vi "Rabi Pulse.vi"() -> ()   [LabVIEW 2012]
uses:
  <vilib>/DAQmx/read.llb/DAQmx Read (Digital Bool 1Line 1Point).vi
  <vilib>/Utility/file.llb/Write To Spreadsheet File (DBL).vi
  <vilib>/DAQmx/create/channels.llb/DAQmx Create Channel (DI-Digital Input).vi
  <vilib>/DAQmx/miscellaneous.llb/DAQmx Fill In Error Info.vi
panel:
  out "Run":bool
  out "size(s)":i32=225
  in  "file path (dialog if empty)":path=path "C:/Users/Ouyang Group/Documents/Data/12-5-13/Rabi pulse sequence 7"
  in  "AOM Pulse length":dbl=3e-07
  in  "N Loop":i32=25000
  in  "Path to spinapi.dll":path=path "C:/SpinCore/SpinAPI/dll/spinapi64.dll"
  in  "stop":bool
  in  "start/restart":bool
  in  "MW width Max":dbl=5e-07
  in  "MW width step size":dbl=2e-09
  in  "MW width Min":dbl=5e-08
  in  "clock_freq (MHz)":dbl=300.0
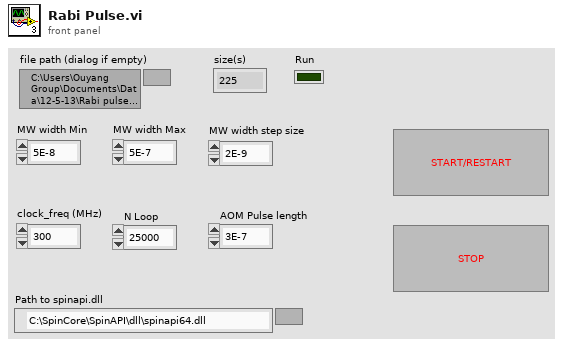
[diagram p1: front panel]
types:
  T1 = cluster{"Instruct Data":i32, "Op Code":i32, "Flags":bool[], "Comments":string, "Time (s)":dbl}
  T2 = enum16{"Pulse Program", "Frequency Registers", "TX Phase Registers", "RX Phase Registers"}
  T3 = cluster{"Instruct Data":i32, "Op Code":i32, "Flags":bool[], "Comments":string, "Time (s)":dbl}[]
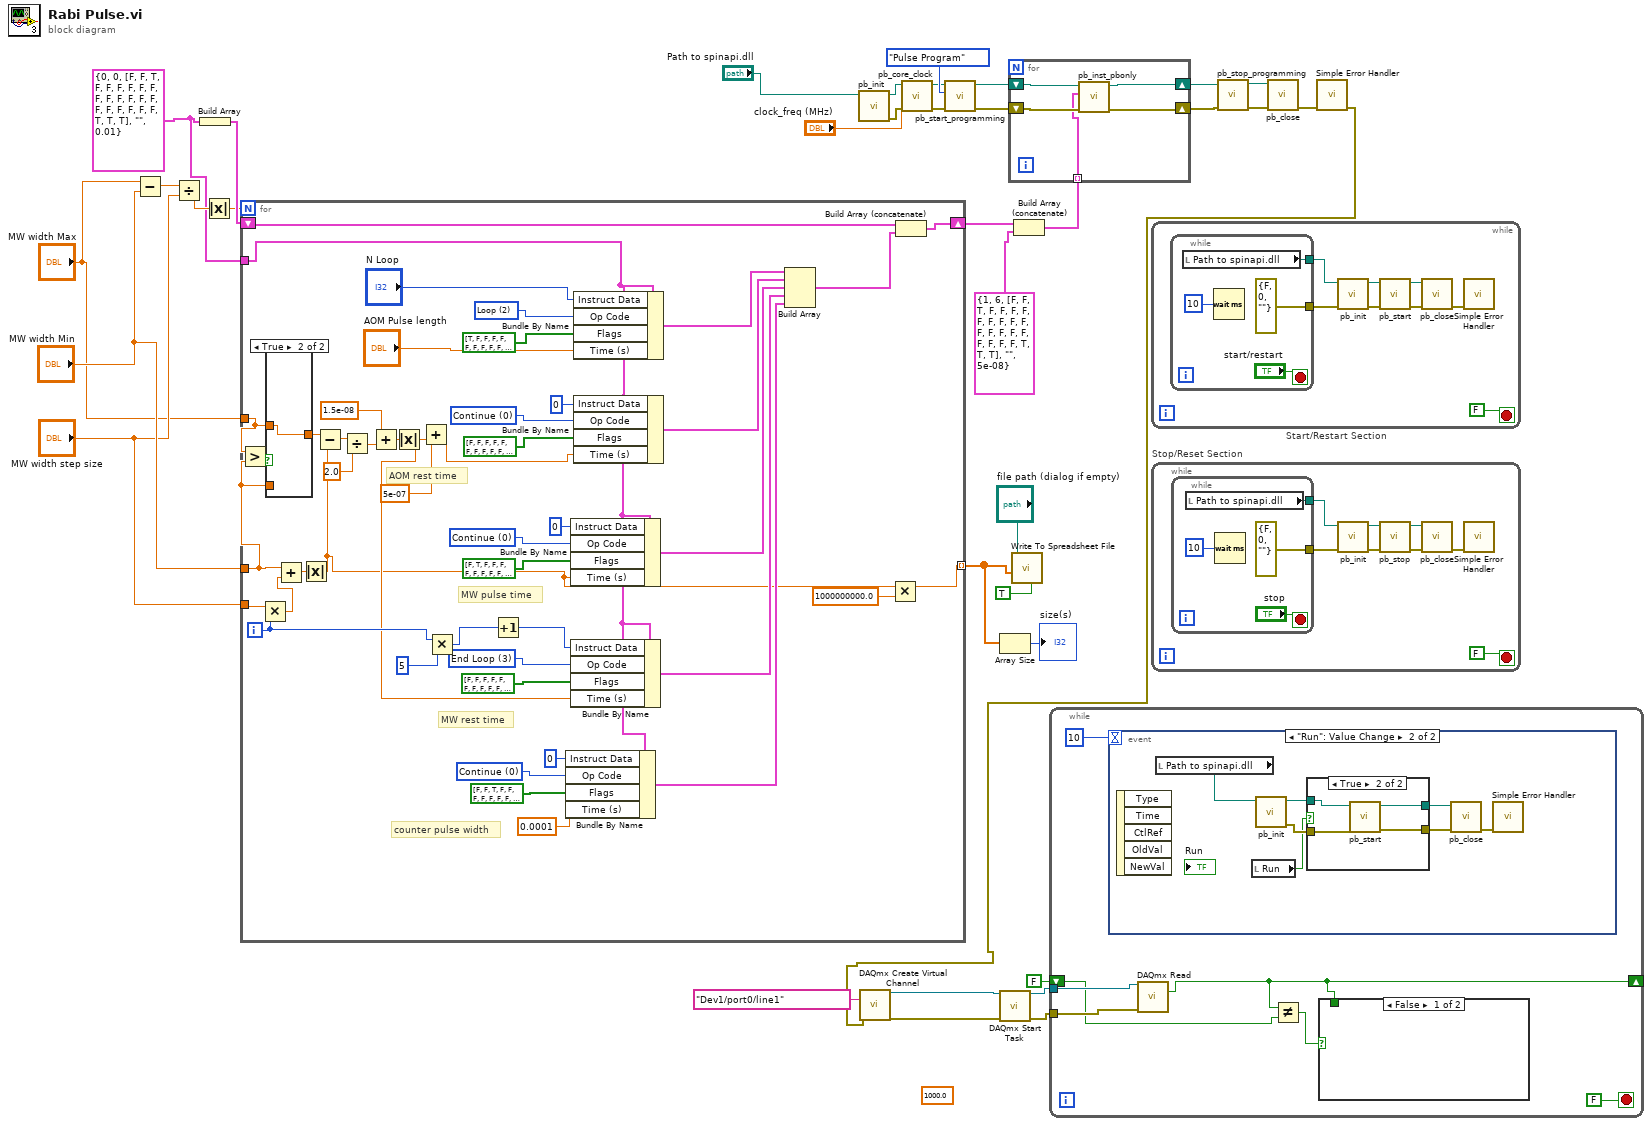
[diagram p0: block diagram]
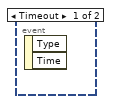
[diagram p2: hidden frame]
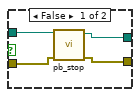
[diagram p3: hidden frame]
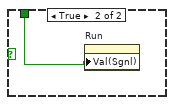
[diagram p4: hidden frame]
diagram:
  (unwired) 1000.0 ("rate")
  w20 = T1 {"Instruct Data"=0, "Op Code"=0, "Flags"=[FALSE, FALSE, TRUE, FALSE, FALSE, FALSE, FALSE, FALSE, FALSE, FALSE, FALSE, FALSE, FALSE, FALSE, FALSE, FALSE, FALSE, FALSE, FALSE, FALSE, FALSE, TRUE, TRUE, TRUE], "Comments"="", "Time (s)"=0.01} ("PB Inst 2")
  n1 = Subtract(x="MW width Max", y="MW width Min") -> (x-y=w24:dbl)
  n2 = Divide(x=w24, y="MW width step size") -> (x/y=w23:dbl)
  n3 = Build Array(w20) -> (w19:T3)
  n4 = Absolute Value(x=w23) -> (abs(x)=w1:dbl)
  n5 = for {
    N: w1 -> [_]
    tunnel: "MW width Min" -> [w39]
    tunnel: "MW width step size" -> [w83]
    tunnel: [w52] -> w11 mode=indexing
    tunnel: w20 -> [w56]
    shift-right: [w80] -> w18
    shift-left: w19 -> [w81]
    tunnel: "MW width Max" -> [w40]
    i -> [w53]
    w67 = 0 items=["Continue", "Stop", "Loop", "End Loop", "JSR", "RTS", "Branch", "Long Delay", "Wait"] ("Op Code")
    w69 = 3 items=["Continue", "Stop", "Loop", "End Loop", "JSR", "RTS", "Branch", "Long Delay", "Wait"] ("Op Code")
    w72 = 0 items=["Continue", "Stop", "Loop", "End Loop", "JSR", "RTS", "Branch", "Long Delay", "Wait"] ("Op Code")
    w75 = 0 items=["Continue", "Stop", "Loop", "End Loop", "JSR", "RTS", "Branch", "Long Delay", "Wait"] ("Op Code")
    w78 = 2 items=["Continue", "Stop", "Loop", "End Loop", "JSR", "RTS", "Branch", "Long Delay", "Wait"] ("Op Code")
    # "counter pulse width"
    # "MW rest time"
    # "MW pulse time"
    # "AOM rest time"
    n6 = Greater?(x=w40, y=w39) -> (0:w42:bool)
    n7 = Multiply(x=w83, y=w53) -> (x*y=w82:dbl)
    n8 = case shown="True" w42 {
      tunnel: [w84 w85] -> w41
      tunnel: w40 -> [_ w85]
      tunnel: w39 -> [w84 _]
      frame False {
      }
      frame True {
      }
    }
    n9 = Add(x=w39, y=w82) -> (x+y=w50:dbl)
    n10 = Absolute Value(x=w50) -> (abs(x)=w43:dbl)
    n11 = Subtract(x=w41, y=w43) -> (x-y=w49:dbl)
    n12 = Divide(x=w49, y=2.0) -> (x/y=w47:dbl)
    n13 = Add(x=1.5e-08, y=w47) -> (x+y=w45:dbl)
    n14 = Absolute Value(x=w45) -> (abs(x)=w44:dbl)
    n15 = Add(x=5e-07, y=w44) -> (x+y=w38:dbl)
    n16 = Multiply(x=w53, y=5) -> (x*y=w54:i32)
    n17 = Increment(x=w54) -> (x+1=w57:i32)
    n18 = Bundle By Name(cluster=w56, "Instruct Data"=0, "Op Code"=w67, "Flags"=bool[] [FALSE, FALSE, TRUE, FALSE, FALSE, FALSE, FALSE, FALSE, FALSE, FALSE, FALSE, FALSE, FALSE, FALSE, FALSE, FALSE, FALSE, FALSE, FALSE, FALSE, FALSE, TRUE, TRUE, TRUE], "Time (s)"=0.0001) -> (w60:T1)
    n19 = Bundle By Name(cluster=w56, "Instruct Data"=0, "Op Code"=w72, "Flags"=bool[] [FALSE, TRUE, FALSE, FALSE, FALSE, FALSE, FALSE, FALSE, FALSE, FALSE, FALSE, FALSE, FALSE, FALSE, FALSE, FALSE, FALSE, FALSE, FALSE, FALSE, FALSE, TRUE, TRUE, TRUE], "Time (s)"=w43) -> (w62:T1)
    n20 = Bundle By Name(cluster=w56, "Instruct Data"=w57, "Op Code"=w69, "Flags"=bool[] [FALSE, FALSE, FALSE, FALSE, FALSE, FALSE, FALSE, FALSE, FALSE, FALSE, FALSE, FALSE, FALSE, FALSE, FALSE, FALSE, FALSE, FALSE, FALSE, FALSE, FALSE, TRUE, TRUE, TRUE], "Time (s)"=w44) -> (w61:T1)
    n21 = Bundle By Name(cluster=w56, "Instruct Data"="N Loop", "Op Code"=w78, "Flags"=bool[] [TRUE, FALSE, FALSE, FALSE, FALSE, FALSE, FALSE, FALSE, FALSE, FALSE, FALSE, FALSE, FALSE, FALSE, FALSE, FALSE, FALSE, FALSE, FALSE, FALSE, FALSE, TRUE, TRUE, TRUE], "Time (s)"="AOM Pulse length") -> (w64:T1)
    n22 = Bundle By Name(cluster=w56, "Instruct Data"=0, "Op Code"=w75, "Flags"=bool[] [FALSE, FALSE, FALSE, FALSE, FALSE, FALSE, FALSE, FALSE, FALSE, FALSE, FALSE, FALSE, FALSE, FALSE, FALSE, FALSE, FALSE, FALSE, FALSE, FALSE, FALSE, TRUE, TRUE, TRUE], "Time (s)"=w38) -> (w63:T1)
    n23 = Build Array(w64, w63, w62, w61, w60) -> (w55:T3)
    n24 = Multiply(x=w43, y=1000000000.0) -> (x*y=w52:dbl)
    n25 = Build Array (concatenate)(w81, w55) -> (w80:T3)
  }
  n26 = call "pb_init.vi"("path in"="Path to spinapi.dll") -> ("error out"=w31:errorcluster, "path out"=w33:path)  [unwired: 3 in, 6 out]
  n27 = call "pb_core_clock.vi"("error in (no error)"=w31, "clock_freq (MHz)"="clock_freq (MHz)", "path in"=w33) -> ("error out"=w30:errorcluster, "path out"=w32:path)  [unwired: 7 in]
  n28 = call "pb_start_programming.vi"("error in (no error)"=w30, "Device"=T2."Pulse Program", "path in"=w32) -> ("error out"=w27:errorcluster, "path out"=w28:path)  [unwired: 1 in, 6 out]
  n29 = Array Size(array=w11) -> (size(s)=→"size(s)":i32)
  n30 = call-poly <vilib>:"Write To Spreadsheet File.vi"("transpose? (no:F)"=TRUE, "1D data"=w11, "file path (dialog if empty)"="file path (dialog if empty)") -> ()  [unwired: 5 in, 1 out]
  n31 = Build Array (concatenate)(w18, T1 {"Instruct Data"=1, "Op Code"=6, "Flags"=[FALSE, FALSE, TRUE, FALSE, FALSE, FALSE, FALSE, FALSE, FALSE, FALSE, FALSE, FALSE, FALSE, FALSE, FALSE, FALSE, FALSE, FALSE, FALSE, FALSE, FALSE, TRUE, TRUE, TRUE], "Comments"="", "Time (s)"=5e-08} ("PB Inst 2")) -> (w17:T3)
  n32 = for {
    tunnel: w17 -> [w86] mode=indexing
    shift-right: [w88] -> w26
    shift-left: w28 -> [w90]
    shift-right: [w87] -> w25
    shift-left: w27 -> [w89]
    n33 = call "pb_inst_pbonly.vi"("error in (no error)"=w89, "PB Instruction"=w86, "path in"=w90) -> ("error out"=w87:errorcluster, "path out"=w88:path)  [unwired: 2 in, 5 out]
  }
  n34 = while "Start/Restart Section" {
    stop <- FALSE stop-if-true
    n35 = while {
      tunnel: [errorcluster {"status"=FALSE, "code"=0, "source"=""} ("error in (no error)")] -> w95
      tunnel: [w99] -> w91
      stop <- "start/restart" stop-if-true
      n36 = local read "Path to spinapi.dll"() -> (w99:path)
      n37 = Wait (ms)(milliseconds to wait=u32 10) -> ()  [unwired: 1 out]
    }
    n38 = call "pb_init.vi"("error in (no error)"=w95, "path in"=w91) -> ("error out"=w94:errorcluster, "path out"=w97:path)  [unwired: 1 in, 7 out]
    n39 = call "pb_start.vi"("error in (no error)"=w94, "path in"=w97) -> ("error out"=w93:errorcluster, "path out"=w98:path)  [unwired: 1 in, 7 out]
    n40 = call "pb_close.vi"("error in (no error)"=w93, "path in"=w98) -> ("error out"=w92:errorcluster)  [unwired: 9 out]
    n41 = call <vilib>:"Simple Error Handler.vi"("error in (no error)"=w92) -> ()  [unwired: 1 in, 8 out]
  }
  n42 = while "Stop/Reset Section" {
    stop <- FALSE stop-if-true
    n43 = while {
      tunnel: [errorcluster {"status"=FALSE, "code"=0, "source"=""} ("error in (no error)")] -> w107
      tunnel: [w111] -> w103
      stop <- "stop" stop-if-true
      n44 = local read "Path to spinapi.dll"() -> (w111:path)
      n45 = Wait (ms)(milliseconds to wait=u32 10) -> ()  [unwired: 1 out]
    }
    n46 = call "pb_init.vi"("error in (no error)"=w107, "path in"=w103) -> ("error out"=w106:errorcluster, "path out"=w109:path)  [unwired: 1 in, 7 out]
    n47 = call "pb_stop.vi"("error in (no error)"=w106, "path in"=w109) -> ("error out"=w105:errorcluster, "path out"=w110:path)  [unwired: 8 out]
    n48 = call "pb_close.vi"("error in (no error)"=w105, "path in"=w110) -> ("error out"=w104:errorcluster)  [unwired: 9 out]
    n49 = call <vilib>:"Simple Error Handler.vi"("error in (no error)"=w104) -> ()  [unwired: 1 in, 8 out]
  }
  n50 = call "pb_stop_programming.vi"("error in (no error)"=w25, "path in"=w26) -> ("error out"=w34:errorcluster, "path out"=w35:path)  [unwired: 1 in, 7 out]
  n51 = call "pb_close.vi"("error in (no error)"=w34, "path in"=w35) -> ("error out"=w14:errorcluster)  [unwired: 9 out]
  n52 = call <vilib>:"Simple Error Handler.vi"("error in (no error)"=w14) -> ("error out"=w5:errorcluster)  [unwired: 1 in, 7 out]
  n53 = call-poly <vilib>:"DAQmx Create Virtual Channel.vi"("lines"=tag "Dev1/port0/line1", "error in"=w5) -> ("task out"=w3:refnum<k21>, "error out"=w2:errorcluster)  [unwired: 12 in]
  n54 = call <vilib>:"DAQmx Start Task.vi"("task/channels in"=w3, "error in"=w2) -> ("task out"=w4:refnum<k21>, "error out"=w7:errorcluster)  [unwired: 12 in]
  n55 = while {
    tunnel: w4 -> [w121]
    tunnel: w7 -> [w120]
    shift-right: [w117] -> _
    shift-left: FALSE ("data") -> [w119]
    stop <- FALSE stop-if-true
    n56 = event shown="[1] \"Run\": Value Change" {
      selector: _ -> [_ _]
      dyn-events: _ -> [_ _]
      timeout: 10 -> [_ _]
      event Timeout {
        n57 = event-data() -> ()  [unwired: 1 in, 2 out]
      }
      event "Run": Value Change {
        n58 = event-data() -> ()  [unwired: 1 in, 5 out]
        n59 = local read "Path to spinapi.dll"() -> (w122:path)
        n60 = local read "Run"() -> (w126:bool)
        n61 = call "pb_init.vi"("path in"=w122) -> ("error out"=w127:errorcluster, "path out"=w128:path)  [unwired: 2 in, 7 out]
        n62 = case shown="True" w126 {
          tunnel: w128 -> [w132 w136]
          tunnel: w127 -> [w131 w135]
          tunnel: [w130 w134] -> w124
          tunnel: [w129 w133] -> w123
          frame False {
            n63 = call "pb_stop.vi"("error in (no error)"=w131, "path in"=w132) -> ("error out"=w129:errorcluster, "path out"=w130:path)  [unwired: 8 out]
          }
          frame True {
            n64 = call "pb_start.vi"("error in (no error)"=w135, "path in"=w136) -> ("error out"=w133:errorcluster, "path out"=w134:path)  [unwired: 1 in, 7 out]
          }
        }
        n65 = call "pb_close.vi"("error in (no error)"=w123, "path in"=w124) -> ("error out"=w125:errorcluster)  [unwired: 9 out]
        n66 = call <vilib>:"Simple Error Handler.vi"("error in (no error)"=w125) -> ()  [unwired: 1 in, 8 out]
      }
    }
    n67 = call-poly <vilib>:"DAQmx Read.vi"("task/channels in"=w121, "error in"=w120) -> ("data"=w117:bool)  [unwired: 11 in, 2 out]
    n68 = Not Equal?(x=w117, y=w119) -> (x != y?=w118:bool)
    n69 = case shown="False" w118 {
      tunnel: w117 -> [_ w137]
      frame False {
      }
      frame True {
        n70 = property on="Run" class="Bool (strict)"("Val(Sgnl)"=w137) -> ()  [unwired: 2 in, 2 out]
      }
    }
  }
